vi "Configure Sequence Pattern.vi"(0 "VISA resource name":refnum<visa-resource-name>, 1 "Pattern (0:Pattern 1)":u16(ring) items=["Pattern 1", "Pattern 2"], 7 "Pattern Mask (0)":i32, 9 "Pattern Value (0)":i32, 11 "error in (no error)":errorcluster) -> (4 "VISA resource name out":refnum<visa-resource-name>, 15 "error out":errorcluster)   [LabVIEW 2017, in "Agilent 6000 Series.lvlib"]
doc: "This VI configures the Sequence trigger. You specify the sequence pattern with the Pattern, Data Value and Data Mask parameters.\n\n<B>NOTE:</B>\n\nThis VI is only valid for 6000 Series models. An error will be thrown if this VI is run with 5000 Series scopes."
uses:
  <instrlib>/Agilent 6000 Series/Agilent 6000 Series.lvlib
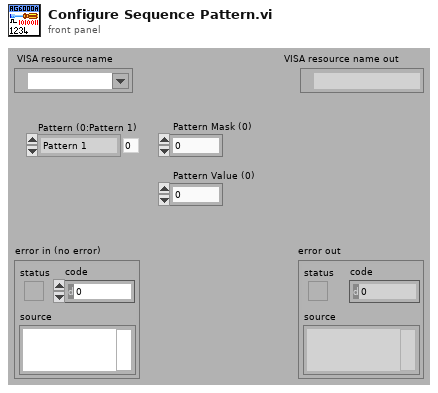
[diagram p1: front panel]
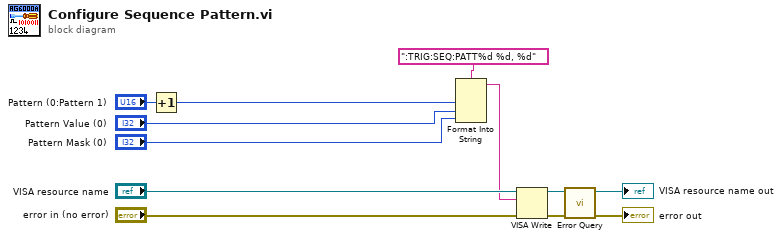
[diagram p0: block diagram]
diagram:
  n1 = Increment(x="Pattern (0:Pattern 1)") -> (x+1=w3:u16)
  n2 = Format Into String(format string=":TRIG:SEQ:PATT%d %d, %d" ("Source Command"), w3, "Pattern Value (0)", "Pattern Mask (0)") -> (resulting string=w5:string)  [unwired: 2 in, 1 out]
  n3 = VISA Write(VISA resource name="VISA resource name", write buffer=w5, error in (no error)="error in (no error)") -> (VISA resource name out=w8:refnum<visa-resource-name>, error out=w7:errorcluster)  [unwired: 1 out]
  n4 = call <instrlib>:"Error Query.vi"("error in (no error)"=w7, "VISA resource name"=w8) -> ("error out"=→"error out":errorcluster, "VISA resource name out"=→"VISA resource name out":refnum<visa-resource-name>)  [unwired: 6 in, 2 out]
